vi "DistributeOutput.vi"(7 "启用输出通道数":T1, 8 "4个通道输出":T2, 9 "2个通道输出":cluster{"AO2":dbl, "AO3 ":dbl}, 10 "一个通道输出AO1":cluster{"AO1":dbl}, 11 "一个通道输出AO0":cluster{"AO0":dbl}) -> (2 "输出数组":dbl[](array[numeric]))   [LabVIEW 2018]
uses:
  Ctl/AO Channel.ctl
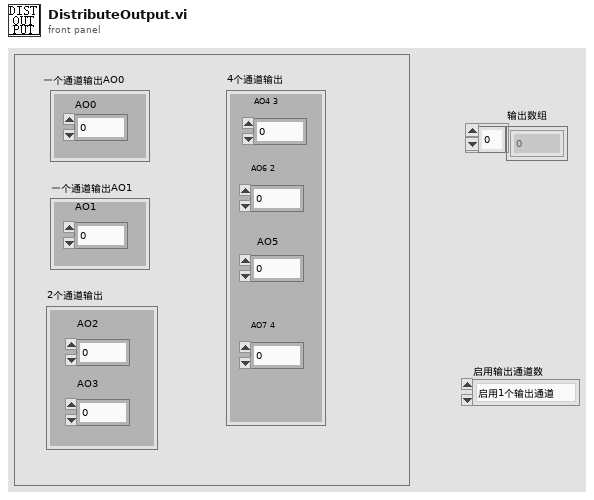
[diagram p1: front panel]
types:
  T1 = typedef "AO Channel.ctl" = enum16{"启用1个输出通道", "启用2个输出通道", "启用3个输出通道", "启用4个输出通道", "启用5个输出通道", "启用6个输出通道", "启用7个输出通道", "启用8个输出通道"}
  T2 = cluster{"AO5":dbl, "AO6 2":dbl, "AO4 3":dbl, "AO7 4":dbl}
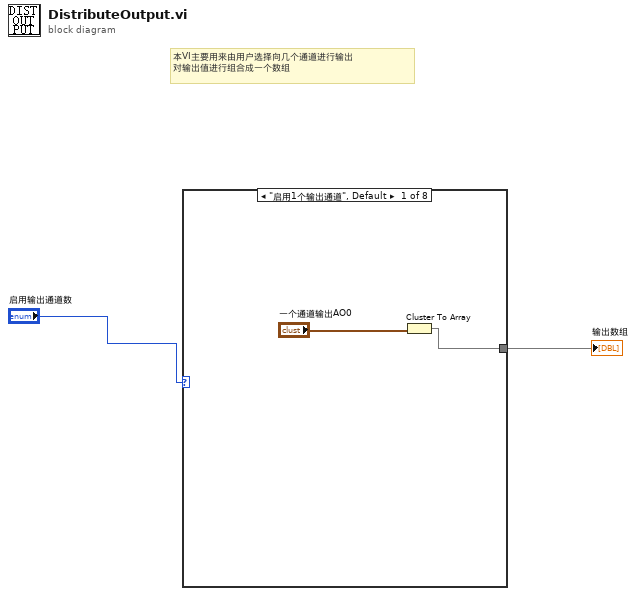
[diagram p0: block diagram]
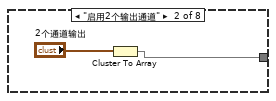
[diagram p2: hidden frame]
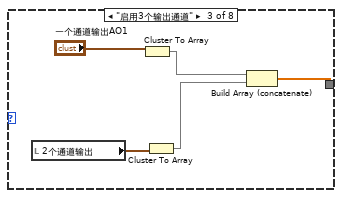
[diagram p3: hidden frame]
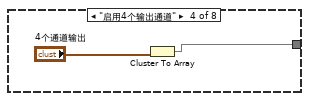
[diagram p4: hidden frame]
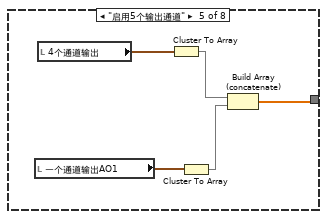
[diagram p5: hidden frame]
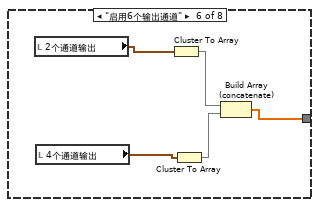
[diagram p6: hidden frame]
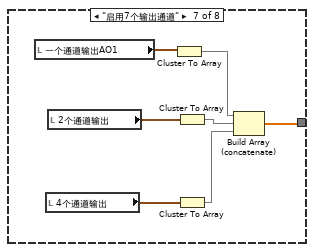
[diagram p7: hidden frame]
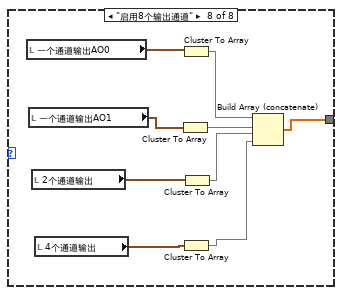
[diagram p8: hidden frame]
diagram:
  # "本VI主要用来由用户选择向几个通道进行输出\n对输出值进行组合成一个数组"
  n1 = case shown="\"启用1个输出通道\", Default" "启用输出通道数" {
    tunnel: [w3 w5 w11 w12 w14 w19 w24 w31] -> w1
    frame "启用1个输出通道", Default {
      n2 = Cluster To Array(cluster="一个通道输出AO0") -> (array=w3:dbl[])
    }
    frame "启用2个输出通道" {
      n3 = Cluster To Array(cluster="2个通道输出") -> (array=w5:dbl[])
    }
    frame "启用3个输出通道" {
      n4 = local read "2个通道输出"() -> (w9:cluster{"AO2":dbl, "AO3 ":dbl})
      n5 = Cluster To Array(cluster="一个通道输出AO1") -> (array=w8:dbl[])
      n6 = Cluster To Array(cluster=w9) -> (array=w7:dbl[])
      n7 = Build Array (concatenate)(w8, w7) -> (w11:dbl[])
    }
    frame "启用4个输出通道" {
      n8 = Cluster To Array(cluster="4个通道输出") -> (array=w12:dbl[])
    }
    frame "启用5个输出通道" {
      n9 = local read "一个通道输出AO1"() -> (w17:cluster{"AO1":dbl})
      n10 = local read "4个通道输出"() -> (w18:T2)
      n11 = Cluster To Array(cluster=w18) -> (array=w16:dbl[])
      n12 = Cluster To Array(cluster=w17) -> (array=w15:dbl[])
      n13 = Build Array (concatenate)(w16, w15) -> (w14:dbl[])
    }
    frame "启用6个输出通道" {
      n14 = local read "2个通道输出"() -> (w23:cluster{"AO2":dbl, "AO3 ":dbl})
      n15 = local read "4个通道输出"() -> (w22:T2)
      n16 = Cluster To Array(cluster=w23) -> (array=w21:dbl[])
      n17 = Cluster To Array(cluster=w22) -> (array=w20:dbl[])
      n18 = Build Array (concatenate)(w21, w20) -> (w19:dbl[])
    }
    frame "启用7个输出通道" {
      n19 = local read "一个通道输出AO1"() -> (w30:cluster{"AO1":dbl})
      n20 = local read "4个通道输出"() -> (w28:T2)
      n21 = local read "2个通道输出"() -> (w29:cluster{"AO2":dbl, "AO3 ":dbl})
      n22 = Cluster To Array(cluster=w30) -> (array=w27:dbl[])
      n23 = Cluster To Array(cluster=w29) -> (array=w26:dbl[])
      n24 = Cluster To Array(cluster=w28) -> (array=w25:dbl[])
      n25 = Build Array (concatenate)(w27, w26, w25) -> (w24:dbl[])
    }
    frame "启用8个输出通道" {
      n26 = local read "一个通道输出AO0"() -> (w39:cluster{"AO0":dbl})
      n27 = local read "一个通道输出AO1"() -> (w38:cluster{"AO1":dbl})
      n28 = local read "2个通道输出"() -> (w37:cluster{"AO2":dbl, "AO3 ":dbl})
      n29 = local read "4个通道输出"() -> (w36:T2)
      n30 = Cluster To Array(cluster=w38) -> (array=w34:dbl[])
      n31 = Cluster To Array(cluster=w39) -> (array=w35:dbl[])
      n32 = Cluster To Array(cluster=w36) -> (array=w32:dbl[])
      n33 = Cluster To Array(cluster=w37) -> (array=w33:dbl[])
      n34 = Build Array (concatenate)(w35, w34, w33, w32) -> (w31:dbl[])
    }
  }
  "输出数组" <- w1
